vi "メイン.vi"() -> (2 "測定周期/ms":dbl, 3 "値転記用配列":T2[](array[typedef]))   [LabVIEW 2021] (continued)
                                w445 = FALSE
                                n187 = property on="メイン測定ボタン_単発 1" class="Bool (指定)"("Visible"=w445) -> ()  [unwired: 2 in, 2 out]
                                n188 = property on="メイン測定ボタン_連続 1" class="Bool (指定)"("Visible"=w445) -> ()  [unwired: 2 in, 2 out]
                              }
                              frame True {
                              }
                            }
                            n189 = local read "メインON/OFF_\n設定 1"() -> (w442:T1)
                            n190 = local write "メインON/OFF_\n保存確認 1"(w442) -> ()
                            n191 = local write "メインON/OFF_制御器 1"(w442) -> ()
                            n192 = property on="メインON/OFF_制御器" class="Clust (指定)"("Visible"=w439) -> ()  [unwired: 2 in, 2 out]
                            n193 = property on="メイン設定No_設定" class="Clust (指定)"("Visible"=w439) -> ()  [unwired: 2 in, 2 out]
                            n194 = property on="メイン設定_設定" class="Clust (指定)"("Visible"=w439) -> ()  [unwired: 2 in, 2 out]
                            n195 = property on="キャンセルボタン" class="Bool (指定)"("Visible"=w439) -> ()  [unwired: 2 in, 2 out]
                          }
                        }
                        n196 = global write "測定キャンセルボタン.vi" "グローバル_測定キャンセルボタン"(w98) -> ()
                        n197 = local write "G_メイン測定キャンセルボタン"(w98) -> ()
                        n198 = local write "測定旧値 1"(w98) -> ()
                        n199 = local write "測定新値 1"(w98) -> ()
                        n200 = control-ref of="このVI"() -> (w95:refnum<vi>)
                        n201 = Unbundle(w97) -> ("Vertical"=w96:i16)  [unwired: 1 out]
                        n202 = Replace Array Subset(array=w101, new element=w100, index=0) -> (w102:T2[])
                        n203 = property on="ペーン 2" class="Pane"("Origin"=w97) -> ()  [unwired: 2 in, 2 out]
                        n204 = call "メイン_装飾移動サブ.vi"("Y軸座標入力"=w96, "VI入力"=w95) -> ()  [unwired: 10 in]
                      }
                    }
                  }
                }
                frame 1 {
                  # "⑱"
                  # "⑰"
                  # "2つ目の配列に転記"
                  # "32回繰り返す為、増やす場合はこのケースストラクチャーを複製する\n複製時、設定項目の配列やボタンも複製する為、下記のボタン類の移動はしない事"
                  # "iniからデータ読み取り"
                  n205 = flat-sequence {
                    tunnel: w456 -> [w482]
                    tunnel: w455 -> [w483]
                    tunnel: [w461] -> w452
                    tunnel: [w460] -> w451
                    tunnel: w452 -> [w629]
                    tunnel: w451 -> [w628]
                    tunnel: [w629] -> w450
                    tunnel: [w628] -> w449
                    tunnel: [w676] -> w457
                    tunnel: [w677] -> w458
                    tunnel: w450 -> [w677]
                    tunnel: w449 -> [w676]
                    tunnel: [w673] -> w447
                    frame #0 {
                      w459 = "設定2"
                      # "複製時に変更する項目\n①②③④⑤⑥⑦⑧⑨　⑪⑫\nローカル変数\n⑬⑭\nセレクション\n⑮⑯\nプロパティノードが\n対象配列になっているか確認\n⑰\n指標値\n⑱\n複製したケースのTrue定数を削除"
                      # "⑭"
                      # "⑬"
                      # "⑫"
                      # "⑪"
                      # "④"
                      # "③"
                      # "setting.iniファイルからの設定項目の読み取り"
                      n206 = local read "メイン設定No_設定 2"() -> (w479:T5)
                      n207 = call-poly <vilib>:"Read Key.vi"("section"="No2.", "error in (no error)"=w483, "key"="No.", "refnum"=w482) -> ("error out"=w476:errorcluster, "value"=w480:i32, "refnum out"=w474:T10)  [unwired: 4 in, 1 out]
                      n208 = Bundle By Name(cluster=w479, "No."=w480) -> (w481:T5)
                      n209 = local write "メイン設定No_設定 2"(w481) -> ()
                      n210 = for {
                        shift-right: [w491] -> w478
                        shift-left: w474 -> [w492]
                        shift-right: [w488] -> w477
                        shift-left: w476 -> [w489]
                        tunnel: string[] ["規格", "規格上限", "規格下限", "ポートNo.", "測定モード", "規格単位", "品質チェック項目", "測定周期", "実測MAX", "実測MIN", "実測(MAX)", "実測(MIN)", "測定画面表示ボタン", "ゲージポートNo."] -> [w487] mode=indexing
                        tunnel: w459 -> [w484]
                        i -> [w490]
                        # "②"
                        # "①"
                        n211 = local read "メイン設定_設定 2"() -> (w485:T2)
                        n212 = case shown="0, デフォルト" w490 {
                          tunnel: w492 -> [w501 w510 w519 w528 w537 w546 w555 w564 w573 w582 w591 w600 w609 w618]
                          tunnel: [w500 w509 w518 w527 w536 w545 w554 w563 w572 w581 w590 w599 w608 w617] -> w491
                          tunnel: w484 -> [w499 w508 w517 w526 w535 w544 w553 w562 w571 w580 w589 w598 w607 w616]
                          tunnel: w489 -> [w498 w507 w516 w525 w534 w543 w552 w561 w570 w579 w588 w597 w606 w615]
                          tunnel: [w497 w506 w515 w524 w533 w542 w551 w560 w569 w578 w587 w596 w605 w614] -> w488
                          tunnel: w487 -> [_ _ _ _ _ w540 _ _ _ _ _ _ _ _]
                          tunnel: w487 -> [_ _ _ _ _ _ w549 _ _ _ _ w594 _ _]
                          tunnel: w487 -> [w495 w504 w513 w522 w531 _ _ w558 w567 w576 w585 _ w603 w612]
                          tunnel: [w494 w503 w512 w521 w530 w538 w547 w556 w566 w575 w584 w593 w602 w611] -> w486
                          tunnel: w485 -> [w493 w502 w511 w520 w529 w539 w548 w557 w565 w574 w583 w592 w601 w610]
                          frame 0, Default {
                            n213 = call-poly <vilib>:"Read Key.vi"("section"=w499, "error in (no error)"=w498, "key"=w495, "refnum"=w501) -> ("error out"=w497:errorcluster, "value"=w496:string, "refnum out"=w500:T10)  [unwired: 4 in, 1 out]
                            n214 = Bundle By Name(cluster=w493, "規格"=w496) -> (w494:T2)
                          }
                          frame 1 {
                            n215 = call-poly <vilib>:"Read Key.vi"("section"=w508, "error in (no error)"=w507, "key"=w504, "refnum"=w510) -> ("error out"=w506:errorcluster, "value"=w505:string, "refnum out"=w509:T10)  [unwired: 4 in, 1 out]
                            n216 = Bundle By Name(cluster=w502, "規格上限"=w505) -> (w503:T2)
                          }
                          frame 2 {
                            n217 = call-poly <vilib>:"Read Key.vi"("section"=w517, "error in (no error)"=w516, "key"=w513, "refnum"=w519) -> ("error out"=w515:errorcluster, "value"=w514:string, "refnum out"=w518:T10)  [unwired: 4 in, 1 out]
                            n218 = Bundle By Name(cluster=w511, "規格下限"=w514) -> (w512:T2)
                          }
                          frame 3 {
                            n219 = call-poly <vilib>:"Read Key.vi"("section"=w526, "error in (no error)"=w525, "key"=w522, "refnum"=w528) -> ("error out"=w524:errorcluster, "value"=w523:i32, "refnum out"=w527:T10)  [unwired: 4 in, 1 out]
                            n220 = Bundle By Name(cluster=w520, "ポートNo."=w523) -> (w521:T2)
                          }
                          frame 4 {
                            n221 = call-poly <vilib>:"Read Key.vi"("section"=w535, "error in (no error)"=w534, "key"=w531, "refnum"=w537) -> ("error out"=w533:errorcluster, "value"=w532:i32, "refnum out"=w536:T10)  [unwired: 4 in, 1 out]
                            n222 = Bundle By Name(cluster=w529, "測定モード"=w532) -> (w530:T2)
                          }
                          frame 5 {
                            n223 = call-poly <vilib>:"Read Key.vi"("section"=w544, "error in (no error)"=w543, "key"=w540, "refnum"=w546) -> ("error out"=w542:errorcluster, "value"=w541:string, "refnum out"=w545:T10)  [unwired: 4 in, 1 out]
                            n224 = Bundle By Name(cluster=w539, "規格単位"=w541) -> (w538:T2)
                          }
                          frame 6 {
                            n225 = call-poly <vilib>:"Read Key.vi"("section"=w553, "error in (no error)"=w552, "key"=w549, "refnum"=w555) -> ("error out"=w551:errorcluster, "value"=w550:string, "refnum out"=w554:T10)  [unwired: 4 in, 1 out]
                            n226 = Bundle By Name(cluster=w548, "品質チェック項目"=w550) -> (w547:T2)
                          }
                          frame 7 {
                            n227 = call-poly <vilib>:"Read Key.vi"("section"=w562, "error in (no error)"=w561, "key"=w558, "refnum"=w564) -> ("error out"=w560:errorcluster, "value"=w559:i32, "refnum out"=w563:T10)  [unwired: 4 in, 1 out]
                            n228 = Bundle By Name(cluster=w557, "測定周期"=w559) -> (w556:T2)
                          }
                          frame 8 {
                            n229 = call-poly <vilib>:"Read Key.vi"("section"=w571, "error in (no error)"=w570, "key"=w567, "refnum"=w573) -> ("error out"=w569:errorcluster, "value"=w568:string, "refnum out"=w572:T10)  [unwired: 4 in, 1 out]
                            n230 = Bundle By Name(cluster=w565, "実測値MAX"=w568) -> (w566:T2)
                          }
                          frame 9 {
                            n231 = call-poly <vilib>:"Read Key.vi"("section"=w580, "error in (no error)"=w579, "key"=w576, "refnum"=w582) -> ("error out"=w578:errorcluster, "value"=w577:string, "refnum out"=w581:T10)  [unwired: 4 in, 1 out]
                            n232 = Bundle By Name(cluster=w574, "実測値MIN"=w577) -> (w575:T2)
                          }
                          frame 10 {
                            n233 = call-poly <vilib>:"Read Key.vi"("section"=w589, "error in (no error)"=w588, "key"=w585, "refnum"=w591) -> ("error out"=w587:errorcluster, "value"=w586:string, "refnum out"=w590:T10)  [unwired: 4 in, 1 out]
                            n234 = Bundle By Name(cluster=w583, "実測値(MAX)"=w586) -> (w584:T2)
                          }
                          frame 11 {
                            n235 = call-poly <vilib>:"Read Key.vi"("section"=w598, "error in (no error)"=w597, "key"=w594, "refnum"=w600) -> ("error out"=w596:errorcluster, "value"=w595:string, "refnum out"=w599:T10)  [unwired: 4 in, 1 out]
                            n236 = Bundle By Name(cluster=w592, "実測値(MIN)"=w595) -> (w593:T2)
                          }
                          frame 12 {
                            n237 = call-poly <vilib>:"Read Key.vi"("section"=w607, "error in (no error)"=w606, "key"=w603, "refnum"=w609) -> ("error out"=w605:errorcluster, "value"=w604:bool, "refnum out"=w608:T10)  [unwired: 4 in, 1 out]
                            n238 = Bundle By Name(cluster=w601, "測定画面表示ボタン"=w604) -> (w602:T2)
                          }
                          frame 13 {
                            n239 = call-poly <vilib>:"Read Key.vi"("section"=w616, "error in (no error)"=w615, "key"=w612, "refnum"=w618) -> ("error out"=w614:errorcluster, "value"=w613:string, "refnum out"=w617:T10)  [unwired: 4 in, 1 out]
                            n240 = Bundle By Name(cluster=w610, "ゲージポートNo"=w613) -> (w611:T2)
                          }
                        }
                        n241 = local write "メイン設定_設定 2"(w486) -> ()
                      }
                      n242 = local read "メインON/OFF_\n設定 2"() -> (w470:T1)
                      n243 = call-poly <vilib>:"Read Key.vi"("section"=w459, "error in (no error)"=w477, "key"="使用ON/OFF", "refnum"=w478) -> ("error out"=w465:errorcluster, "value"=w468:bool, "refnum out"=w466:T10)  [unwired: 4 in, 1 out]
                      n244 = Bundle By Name(cluster=w470, "使用ON/OFF"=w468) -> (w471:T1)
                      n245 = local write "メインON/OFF_\n設定 2"(w471) -> ()
                      n246 = local read "CSV項目名 2"() -> (w464:T3)
                      n247 = call-poly <vilib>:"Read Key.vi"("section"=w459, "error in (no error)"=w465, "key"="CSVヘッダー名", "refnum"=w466) -> ("error out"=w460:errorcluster, "value"=w462:string, "refnum out"=w461:T10)  [unwired: 4 in, 1 out]
                      n248 = Bundle By Name(cluster=w464, "CSV項目名"=w462) -> (w463:T3)
                      n249 = local write "CSV項目名 2"(w463) -> ()
                    }
                    frame #1 {
                      # "csvヘッダー項目作成"
                      # "⑮"
                      # "⑤"
                      n250 = local read "CSV項目名 2"() -> (w623:T3)
                      n251 = Unbundle By Name(w623) -> ("CSV項目名"=w620:string)
                      n252 = local read "メイン設定_設定 2"() -> (w624:T2)
                      n253 = Unbundle By Name(w624) -> ("測定モード"=w619:u16)
                      n254 = case shown="0, デフォルト" w619 {
                        tunnel: ["単発測定" _ "多点測定"] -> w627
                        tunnel: [FALSE TRUE FALSE] -> w626
                        tunnel: [TRUE FALSE TRUE] -> w625
                        frame 0, Default {
                        }
                        frame 1 {
                        }
                        frame 2 {
                        }
                      }
                      n255 = case shown="1" w619 {
                        tunnel: w620 -> [w633 w645 w654]
                        tunnel: [w631 w643 w656] -> w622
                        tunnel: [w630 w642 w655] -> w621
                        frame 1 {
                          n256 = Empty String/Path?(string/path=w633) -> (empty?=w632:bool)
                          n257 = case shown="FALSE" w632 {
                            tunnel: w633 -> [w639 _]
                            tunnel: w633 -> [w638 _]
                            tunnel: [w635 ""] -> w631
                            tunnel: [w634 ""] -> w630
                            frame False {
                              n258 = Concatenate Strings(w639, "_max") -> (w635:string)
                              n259 = Concatenate Strings(w638, "_min") -> (w634:string)
                            }
                            frame True {
                            }
                          }
                        }
                        frame 2 {
                          n260 = Empty String/Path?(string/path=w645) -> (empty?=w644:bool)
                          n261 = case shown="FALSE" w644 {
                            tunnel: w645 -> [w651 _]
                            tunnel: w645 -> [w650 _]
                            tunnel: [w647 ""] -> w643
                            tunnel: [w646 ""] -> w642
                            frame False {
                              n262 = Concatenate Strings(w651, "_max") -> (w647:string)
                              n263 = Concatenate Strings(w650, "_min") -> (w646:string)
                            }
                            frame True {
                            }
                          }
                        }
                        frame 0, Default {
                          n264 = Empty String/Path?(string/path=w654) -> (empty?=w657:bool)
                          n265 = case shown="FALSE" w657 {
                            tunnel: w654 -> [w661 _]
                            tunnel: [w659 ""] -> w656
                            tunnel: ["" ""] -> w655
                            frame False {
                              n266 = Concatenate Strings(w661, "_value") -> (w659:string)
                            }
                            frame True {
                            }
                          }
                        }
                      }
                      n267 = property on="メイン測定ボタン_単発 2" class="Bool (指定)"("BoolText.Text"=w627) -> ()  [unwired: 2 in, 2 out]
                      n268 = local write "csv入力項目min 2"(w621) -> ()
                      n269 = local write "csv入力項目max 2"(w622) -> ()
                      n270 = property on="メイン測定ボタン_連続 2" class="Bool (指定)"("Visible"=w626) -> ()  [unwired: 2 in, 2 out]
                      n271 = property on="メイン測定ボタン_単発 2" class="Bool (指定)"("Visible"=w625) -> ()  [unwired: 2 in, 2 out]
                    }
                    frame #2 {
                      # "⑯"
                      # "⑨"
                      # "⑧"
                      # "⑦"
                      # "⑥"
                      n272 = local read "メインON/OFF_\n設定 2"() -> (w675:T1)
                      n273 = local write "メインON/OFF_\n保存確認 2"(w675) -> ()
                      n274 = local read "メイン設定_設定 2"() -> (w673:T2)
                      n275 = Unbundle By Name(w673) -> ("測定画面表示ボタン"=w672:bool)
                      n276 = case shown="FALSE" w672 {
                        tunnel: [w678 TRUE] -> w674
                        frame False {
                          w678 = FALSE
                          n277 = property on="メイン測定ボタン_単発 2" class="Bool (指定)"("Visible"=w678) -> ()  [unwired: 2 in, 2 out]
                          n278 = property on="メイン測定ボタン_連続 2" class="Bool (指定)"("Visible"=w678) -> ()  [unwired: 2 in, 2 out]
                        }
                        frame True {
                        }
                      }
                      n279 = local write "メインON/OFF_制御器 2"(w675) -> ()
                      n280 = property on="メインON/OFF_制御器 2" class="Clust (指定)"("Visible"=w674) -> ()  [unwired: 2 in, 2 out]
                      n281 = property on="メイン設定No_設定 2" class="Clust (指定)"("Visible"=w674) -> ()  [unwired: 2 in, 2 out]
                      n282 = property on="メイン設定_設定 2" class="Clust (指定)"("Visible"=w674) -> ()  [unwired: 2 in, 2 out]
                      n283 = property on="キャンセルボタン 2" class="Bool (指定)"("Visible"=w674) -> ()  [unwired: 2 in, 2 out]
                    }
                  }
                  n284 = Replace Array Subset(array=w454, new element=w447, index=1) -> (w453:T2[])
                }
                frame 2 {
                  # "⑱"
                  # "⑰"
                  # "2つ目の配列に転記"
                  # "32回繰り返す為、増やす場合はこのケースストラクチャーを複製する\n複製時、設定項目の配列やボタンも複製する為、下記のボタン類の移動はしない事"
                  # "iniからデータ読み取り"
                  n285 = flat-sequence {
                    tunnel: w689 -> [w715]
                    tunnel: w688 -> [w716]
                    tunnel: [w693] -> w685
                    tunnel: [w694] -> w684
                    tunnel: w685 -> [w862]
                    tunnel: w684 -> [w861]
                    tunnel: [w862] -> w683
                    tunnel: [w861] -> w682
                    tunnel: [w909] -> w690
                    tunnel: [w910] -> w691
                    tunnel: w683 -> [w910]
                    tunnel: w682 -> [w909]
                    tunnel: [w906] -> w680
                    frame #0 {
                      w692 = "設定3"
                      # "複製時に変更する項目\n①②③④⑤⑥⑦⑧⑨　⑪⑫\nローカル変数\n⑬⑭\nセレクション\n⑮⑯\nプロパティノードが\n対象配列になっているか確認\n⑰\n指標値\n⑱\n複製したケースのTrue定数を削除"
                      # "⑭"
                      # "⑬"
                      # "⑫"
                      # "⑪"
                      # "④"
                      # "③"
                      # "setting.iniファイルからの設定項目の読み取り"
                      n286 = local read "メイン設定No_設定 3"() -> (w712:T5)
                      n287 = call-poly <vilib>:"Read Key.vi"("section"="No3.", "error in (no error)"=w716, "key"="No.", "refnum"=w715) -> ("error out"=w709:errorcluster, "value"=w713:i32, "refnum out"=w707:T10)  [unwired: 4 in, 1 out]
                      n288 = Bundle By Name(cluster=w712, "No."=w713) -> (w714:T5)
                      n289 = local write "メイン設定No_設定 3"(w714) -> ()
                      n290 = for {
                        shift-right: [w724] -> w711
                        shift-left: w707 -> [w725]
                        shift-right: [w721] -> w710
                        shift-left: w709 -> [w722]
                        tunnel: string[] ["規格", "規格上限", "規格下限", "ポートNo.", "測定モード", "規格単位", "品質チェック項目", "測定周期", "実測MAX", "実測MIN", "実測(MAX)", "実測(MIN)", "測定画面表示ボタン", "ゲージポートNo."] -> [w720] mode=indexing
                        tunnel: w692 -> [w717]
                        i -> [w723]
                        # "②"
                        # "①"
                        n291 = local read "メイン設定_設定 3"() -> (w718:T2)
                        n292 = case shown="0, デフォルト" w723 {
                          tunnel: w725 -> [w734 w743 w752 w761 w770 w779 w788 w797 w806 w815 w824 w833 w842 w851]
                          tunnel: [w733 w742 w751 w760 w769 w778 w787 w796 w805 w814 w823 w832 w841 w850] -> w724
                          tunnel: w717 -> [w732 w741 w750 w759 w768 w777 w786 w795 w804 w813 w822 w831 w840 w849]
                          tunnel: w722 -> [w731 w740 w749 w758 w767 w776 w785 w794 w803 w812 w821 w830 w839 w848]
                          tunnel: [w730 w739 w748 w757 w766 w775 w784 w793 w802 w811 w820 w829 w838 w847] -> w721
                          tunnel: w720 -> [_ _ _ _ _ w773 _ _ _ _ _ _ _ _]
                          tunnel: w720 -> [_ _ _ _ _ _ w782 _ _ _ _ w827 _ _]
                          tunnel: w720 -> [w728 w737 w746 w755 w764 _ _ w791 w800 w809 w818 _ w836 w845]
                          tunnel: [w727 w736 w745 w754 w763 w771 w780 w789 w799 w808 w817 w826 w835 w844] -> w719
                          tunnel: w718 -> [w726 w735 w744 w753 w762 w772 w781 w790 w798 w807 w816 w825 w834 w843]
                          frame 0, Default {
                            n293 = call-poly <vilib>:"Read Key.vi"("section"=w732, "error in (no error)"=w731, "key"=w728, "refnum"=w734) -> ("error out"=w730:errorcluster, "value"=w729:string, "refnum out"=w733:T10)  [unwired: 4 in, 1 out]
                            n294 = Bundle By Name(cluster=w726, "規格"=w729) -> (w727:T2)
                          }
                          frame 1 {
                            n295 = call-poly <vilib>:"Read Key.vi"("section"=w741, "error in (no error)"=w740, "key"=w737, "refnum"=w743) -> ("error out"=w739:errorcluster, "value"=w738:string, "refnum out"=w742:T10)  [unwired: 4 in, 1 out]
                            n296 = Bundle By Name(cluster=w735, "規格上限"=w738) -> (w736:T2)
                          }
                          frame 2 {
                            n297 = call-poly <vilib>:"Read Key.vi"("section"=w750, "error in (no error)"=w749, "key"=w746, "refnum"=w752) -> ("error out"=w748:errorcluster, "value"=w747:string, "refnum out"=w751:T10)  [unwired: 4 in, 1 out]
                            n298 = Bundle By Name(cluster=w744, "規格下限"=w747) -> (w745:T2)
                          }
                          frame 3 {
                            n299 = call-poly <vilib>:"Read Key.vi"("section"=w759, "error in (no error)"=w758, "key"=w755, "refnum"=w761) -> ("error out"=w757:errorcluster, "value"=w756:i32, "refnum out"=w760:T10)  [unwired: 4 in, 1 out]
                            n300 = Bundle By Name(cluster=w753, "ポートNo."=w756) -> (w754:T2)
                          }
                          frame 4 {
                            n301 = call-poly <vilib>:"Read Key.vi"("section"=w768, "error in (no error)"=w767, "key"=w764, "refnum"=w770) -> ("error out"=w766:errorcluster, "value"=w765:i32, "refnum out"=w769:T10)  [unwired: 4 in, 1 out]
                            n302 = Bundle By Name(cluster=w762, "測定モード"=w765) -> (w763:T2)
                          }
                          frame 5 {
                            n303 = call-poly <vilib>:"Read Key.vi"("section"=w777, "error in (no error)"=w776, "key"=w773, "refnum"=w779) -> ("error out"=w775:errorcluster, "value"=w774:string, "refnum out"=w778:T10)  [unwired: 4 in, 1 out]
                            n304 = Bundle By Name(cluster=w772, "規格単位"=w774) -> (w771:T2)
                          }
                          frame 6 {
                            n305 = call-poly <vilib>:"Read Key.vi"("section"=w786, "error in (no error)"=w785, "key"=w782, "refnum"=w788) -> ("error out"=w784:errorcluster, "value"=w783:string, "refnum out"=w787:T10)  [unwired: 4 in, 1 out]
                            n306 = Bundle By Name(cluster=w781, "品質チェック項目"=w783) -> (w780:T2)
                          }
                          frame 7 {
                            n307 = call-poly <vilib>:"Read Key.vi"("section"=w795, "error in (no error)"=w794, "key"=w791, "refnum"=w797) -> ("error out"=w793:errorcluster, "value"=w792:i32, "refnum out"=w796:T10)  [unwired: 4 in, 1 out]
                            n308 = Bundle By Name(cluster=w790, "測定周期"=w792) -> (w789:T2)
                          }
                          frame 8 {
                            n309 = call-poly <vilib>:"Read Key.vi"("section"=w804, "error in (no error)"=w803, "key"=w800, "refnum"=w806) -> ("error out"=w802:errorcluster, "value"=w801:string, "refnum out"=w805:T10)  [unwired: 4 in, 1 out]
                            n310 = Bundle By Name(cluster=w798, "実測値MAX"=w801) -> (w799:T2)
                          }
                          frame 9 {
                            n311 = call-poly <vilib>:"Read Key.vi"("section"=w813, "error in (no error)"=w812, "key"=w809, "refnum"=w815) -> ("error out"=w811:errorcluster, "value"=w810:string, "refnum out"=w814:T10)  [unwired: 4 in, 1 out]
                            n312 = Bundle By Name(cluster=w807, "実測値MIN"=w810) -> (w808:T2)
                          }
                          frame 10 {
                            n313 = call-poly <vilib>:"Read Key.vi"("section"=w822, "error in (no error)"=w821, "key"=w818, "refnum"=w824) -> ("error out"=w820:errorcluster, "value"=w819:string, "refnum out"=w823:T10)  [unwired: 4 in, 1 out]
                            n314 = Bundle By Name(cluster=w816, "実測値(MAX)"=w819) -> (w817:T2)
                          }
                          frame 11 {
                            n315 = call-poly <vilib>:"Read Key.vi"("section"=w831, "error in (no error)"=w830, "key"=w827, "refnum"=w833) -> ("error out"=w829:errorcluster, "value"=w828:string, "refnum out"=w832:T10)  [unwired: 4 in, 1 out]
                            n316 = Bundle By Name(cluster=w825, "実測値(MIN)"=w828) -> (w826:T2)
                          }
                          frame 12 {
                            n317 = call-poly <vilib>:"Read Key.vi"("section"=w840, "error in (no error)"=w839, "key"=w836, "refnum"=w842) -> ("error out"=w838:errorcluster, "value"=w837:bool, "refnum out"=w841:T10)  [unwired: 4 in, 1 out]
                            n318 = Bundle By Name(cluster=w834, "測定画面表示ボタン"=w837) -> (w835:T2)
                          }
                          frame 13 {
                            n319 = call-poly <vilib>:"Read Key.vi"("section"=w849, "error in (no error)"=w848, "key"=w845, "refnum"=w851) -> ("error out"=w847:errorcluster, "value"=w846:string, "refnum out"=w850:T10)  [unwired: 4 in, 1 out]
                            n320 = Bundle By Name(cluster=w843, "ゲージポートNo"=w846) -> (w844:T2)
                          }
                        }
                        n321 = local write "メイン設定_設定 3"(w719) -> ()
                      }
                      n322 = local read "メインON/OFF_\n設定 3"() -> (w703:T1)
                      n323 = call-poly <vilib>:"Read Key.vi"("section"=w692, "error in (no error)"=w710, "key"="使用ON/OFF", "refnum"=w711) -> ("error out"=w695:errorcluster, "value"=w701:bool, "refnum out"=w696:T10)  [unwired: 4 in, 1 out]
                      n324 = Bundle By Name(cluster=w703, "使用ON/OFF"=w701) -> (w704:T1)
                      n325 = local write "メインON/OFF_\n設定 3"(w704) -> ()
                      n326 = local read "CSV項目名 3"() -> (w699:T3)
                      n327 = call-poly <vilib>:"Read Key.vi"("section"=w692, "error in (no error)"=w695, "key"="CSVヘッダー名", "refnum"=w696) -> ("error out"=w694:errorcluster, "value"=w697:string, "refnum out"=w693:T10)  [unwired: 4 in, 1 out]
                      n328 = Bundle By Name(cluster=w699, "CSV項目名"=w697) -> (w698:T3)
                      n329 = local write "CSV項目名 3"(w698) -> ()
                    }
                    frame #1 {
                      # "csvヘッダー項目作成"
                      # "⑮"
                      # "⑤"
                      n330 = local read "CSV項目名 3"() -> (w856:T3)
                      n331 = Unbundle By Name(w856) -> ("CSV項目名"=w853:string)
                      n332 = local read "メイン設定_設定 3"() -> (w857:T2)
                      n333 = Unbundle By Name(w857) -> ("測定モード"=w852:u16)
                      n334 = case shown="0, デフォルト" w852 {
                        tunnel: ["単発測定" _ "多点測定"] -> w860
                        tunnel: [FALSE TRUE FALSE] -> w859
                        tunnel: [TRUE FALSE TRUE] -> w858
                        frame 0, Default {
                        }
                        frame 1 {
                        }
                        frame 2 {
                        }
                      }
                      n335 = case shown="1" w852 {
                        tunnel: w853 -> [w866 w878 w887]
                        tunnel: [w864 w876 w889] -> w855
                        tunnel: [w863 w875 w888] -> w854
                        frame 1 {
                          n336 = Empty String/Path?(string/path=w866) -> (empty?=w865:bool)
                          n337 = case shown="FALSE" w865 {
                            tunnel: w866 -> [w872 _]
                            tunnel: w866 -> [w871 _]
                            tunnel: [w868 ""] -> w864
                            tunnel: [w867 ""] -> w863
                            frame False {
                              n338 = Concatenate Strings(w872, "_max") -> (w868:string)
                              n339 = Concatenate Strings(w871, "_min") -> (w867:string)
                            }
                            frame True {
                            }
                          }
                        }
                        frame 2 {
                          n340 = Empty String/Path?(string/path=w878) -> (empty?=w877:bool)
                          n341 = case shown="FALSE" w877 {
                            tunnel: w878 -> [w884 _]
                            tunnel: w878 -> [w883 _]
                            tunnel: [w880 ""] -> w876
                            tunnel: [w879 ""] -> w875
                            frame False {
                              n342 = Concatenate Strings(w884, "_max") -> (w880:string)
                              n343 = Concatenate Strings(w883, "_min") -> (w879:string)
                            }
                            frame True {
                            }
                          }
                        }
                        frame 0, Default {
                          n344 = Empty String/Path?(string/path=w887) -> (empty?=w890:bool)
                          n345 = case shown="FALSE" w890 {
                            tunnel: w887 -> [w894 _]
                            tunnel: [w892 ""] -> w889
                            tunnel: ["" ""] -> w888
                            frame False {
                              n346 = Concatenate Strings(w894, "_value") -> (w892:string)
                            }
                            frame True {
                            }
                          }
                        }
                      }
                      n347 = property on="メイン測定ボタン_単発 3" class="Bool (指定)"("BoolText.Text"=w860) -> ()  [unwired: 2 in, 2 out]
                      n348 = local write "csv入力項目min 3"(w854) -> ()
                      n349 = local write "csv入力項目max 3"(w855) -> ()
                      n350 = property on="メイン測定ボタン_連続 3" class="Bool (指定)"("Visible"=w859) -> ()  [unwired: 2 in, 2 out]
                      n351 = property on="メイン測定ボタン_単発 3" class="Bool (指定)"("Visible"=w858) -> ()  [unwired: 2 in, 2 out]
                    }
                    frame #2 {
                      # "⑯"
                      # "⑨"
                      # "⑧"
                      # "⑦"
                      # "⑥"
                      n352 = local read "メインON/OFF_\n設定 3"() -> (w908:T1)
                      n353 = local write "メインON/OFF_\n保存確認 3"(w908) -> ()
                      n354 = local read "メイン設定_設定 3"() -> (w906:T2)
                      n355 = Unbundle By Name(w906) -> ("測定画面表示ボタン"=w905:bool)
                      n356 = case shown="FALSE" w905 {
                        tunnel: [w911 TRUE] -> w907
                        frame False {
                          w911 = FALSE
                          n357 = property on="メイン測定ボタン_単発 3" class="Bool (指定)"("Visible"=w911) -> ()  [unwired: 2 in, 2 out]
                          n358 = property on="メイン測定ボタン_連続 3" class="Bool (指定)"("Visible"=w911) -> ()  [unwired: 2 in, 2 out]
                        }
                        frame True {
                        }
                      }
                      n359 = local write "メインON/OFF_制御器 3"(w908) -> ()
                      n360 = property on="メインON/OFF_制御器 3" class="Clust (指定)"("Visible"=w907) -> ()  [unwired: 2 in, 2 out]
                      n361 = property on="メイン設定No_設定 3" class="Clust (指定)"("Visible"=w907) -> ()  [unwired: 2 in, 2 out]
                      n362 = property on="メイン設定_設定 3" class="Clust (指定)"("Visible"=w907) -> ()  [unwired: 2 in, 2 out]
                      n363 = property on="キャンセルボタン 3" class="Bool (指定)"("Visible"=w907) -> ()  [unwired: 2 in, 2 out]
                    }
                  }
                  n364 = Replace Array Subset(array=w687, new element=w680, index=2) -> (w686:T2[])
                }
                frame 3 {
                  # "⑱"
                  # "⑰"
                  # "2つ目の配列に転記"
                  # "32回繰り返す為、増やす場合はこのケースストラクチャーを複製する\n複製時、設定項目の配列やボタンも複製する為、下記のボタン類の移動はしない事"
                  # "iniからデータ読み取り"
                  n365 = flat-sequence {
                    tunnel: w922 -> [w948]
                    tunnel: w921 -> [w949]
                    tunnel: [w927] -> w918
                    tunnel: [w926] -> w913
                    tunnel: w918 -> [w1095]
                    tunnel: [w1095] -> w917
                    tunnel: [w1094] -> w916
                    tunnel: w913 -> [w1094]
                    tunnel: [w1142] -> w923
                    tunnel: [w1143] -> w924
                    tunnel: w917 -> [w1143]
                    tunnel: w916 -> [w1142]
                    tunnel: [w1139] -> w914
                    frame #0 {
                      w925 = "設定4"
                      # "複製時に変更する項目\n①②③④⑤⑥⑦⑧⑨　⑪⑫\nローカル変数\n⑬⑭\nセレクション\n⑮⑯\nプロパティノードが\n対象配列になっているか確認\n⑰\n指標値\n⑱\n複製したケースのTrue定数を削除"
                      # "⑭"
                      # "⑬"
                      # "⑫"
                      # "⑪"
                      # "④"
                      # "③"
                      # "setting.iniファイルからの設定項目の読み取り"
                      n366 = local read "メイン設定No_設定 4"() -> (w945:T5)
                      n367 = call-poly <vilib>:"Read Key.vi"("section"="No4.", "error in (no error)"=w949, "key"="No.", "refnum"=w948) -> ("error out"=w942:errorcluster, "value"=w946:i32, "refnum out"=w940:T10)  [unwired: 4 in, 1 out]
                      n368 = Bundle By Name(cluster=w945, "No."=w946) -> (w947:T5)
                      n369 = local write "メイン設定No_設定 4"(w947) -> ()
                      n370 = for {
                        shift-right: [w957] -> w944
                        shift-left: w940 -> [w958]
                        shift-right: [w954] -> w943
                        shift-left: w942 -> [w955]
                        tunnel: string[] ["規格", "規格上限", "規格下限", "ポートNo.", "測定モード", "規格単位", "品質チェック項目", "測定周期", "実測MAX", "実測MIN", "実測(MAX)", "実測(MIN)", "測定画面表示ボタン", "ゲージポートNo."] -> [w953] mode=indexing
                        tunnel: w925 -> [w950]
                        i -> [w956]
                        # "②"
                        # "①"
                        n371 = local read "メイン設定_設定 4"() -> (w951:T2)
                        n372 = case shown="0, デフォルト" w956 {
                          tunnel: w958 -> [w967 w976 w985 w994 w1003 w1012 w1021 w1030 w1039 w1048 w1057 w1066 w1075 w1084]
                          tunnel: [w966 w975 w984 w993 w1002 w1011 w1020 w1029 w1038 w1047 w1056 w1065 w1074 w1083] -> w957
                          tunnel: w950 -> [w965 w974 w983 w992 w1001 w1010 w1019 w1028 w1037 w1046 w1055 w1064 w1073 w1082]
                          tunnel: w955 -> [w964 w973 w982 w991 w1000 w1009 w1018 w1027 w1036 w1045 w1054 w1063 w1072 w1081]
                          tunnel: [w963 w972 w981 w990 w999 w1008 w1017 w1026 w1035 w1044 w1053 w1062 w1071 w1080] -> w954
                          tunnel: w953 -> [_ _ _ _ _ w1006 _ _ _ _ _ _ _ _]
                          tunnel: w953 -> [_ _ _ _ _ _ w1015 _ _ _ _ w1060 _ _]
                          tunnel: w953 -> [w961 w970 w979 w988 w997 _ _ w1024 w1033 w1042 w1051 _ w1069 w1078]
                          tunnel: [w960 w969 w978 w987 w996 w1004 w1013 w1022 w1032 w1041 w1050 w1059 w1068 w1077] -> w952
                          tunnel: w951 -> [w959 w968 w977 w986 w995 w1005 w1014 w1023 w1031 w1040 w1049 w1058 w1067 w1076]
                          frame 0, Default {
                            n373 = call-poly <vilib>:"Read Key.vi"("section"=w965, "error in (no error)"=w964, "key"=w961, "refnum"=w967) -> ("error out"=w963:errorcluster, "value"=w962:string, "refnum out"=w966:T10)  [unwired: 4 in, 1 out]
                            n374 = Bundle By Name(cluster=w959, "規格"=w962) -> (w960:T2)
                          }
                          frame 1 {
                            n375 = call-poly <vilib>:"Read Key.vi"("section"=w974, "error in (no error)"=w973, "key"=w970, "refnum"=w976) -> ("error out"=w972:errorcluster, "value"=w971:string, "refnum out"=w975:T10)  [unwired: 4 in, 1 out]
                            n376 = Bundle By Name(cluster=w968, "規格上限"=w971) -> (w969:T2)
                          }
                          frame 2 {
                            n377 = call-poly <vilib>:"Read Key.vi"("section"=w983, "error in (no error)"=w982, "key"=w979, "refnum"=w985) -> ("error out"=w981:errorcluster, "value"=w980:string, "refnum out"=w984:T10)  [unwired: 4 in, 1 out]
                            n378 = Bundle By Name(cluster=w977, "規格下限"=w980) -> (w978:T2)
                          }
                          frame 3 {
                            n379 = call-poly <vilib>:"Read Key.vi"("section"=w992, "error in (no error)"=w991, "key"=w988, "refnum"=w994) -> ("error out"=w990:errorcluster, "value"=w989:i32, "refnum out"=w993:T10)  [unwired: 4 in, 1 out]
                            n380 = Bundle By Name(cluster=w986, "ポートNo."=w989) -> (w987:T2)
                          }
                          frame 4 {
                            n381 = call-poly <vilib>:"Read Key.vi"("section"=w1001, "error in (no error)"=w1000, "key"=w997, "refnum"=w1003) -> ("error out"=w999:errorcluster, "value"=w998:i32, "refnum out"=w1002:T10)  [unwired: 4 in, 1 out]
                            n382 = Bundle By Name(cluster=w995, "測定モード"=w998) -> (w996:T2)
                          }
                          frame 5 {
                            n383 = call-poly <vilib>:"Read Key.vi"("section"=w1010, "error in (no error)"=w1009, "key"=w1006, "refnum"=w1012) -> ("error out"=w1008:errorcluster, "value"=w1007:string, "refnum out"=w1011:T10)  [unwired: 4 in, 1 out]
                            n384 = Bundle By Name(cluster=w1005, "規格単位"=w1007) -> (w1004:T2)
                          }
                          frame 6 {
                            n385 = call-poly <vilib>:"Read Key.vi"("section"=w1019, "error in (no error)"=w1018, "key"=w1015, "refnum"=w1021) -> ("error out"=w1017:errorcluster, "value"=w1016:string, "refnum out"=w1020:T10)  [unwired: 4 in, 1 out]
                            n386 = Bundle By Name(cluster=w1014, "品質チェック項目"=w1016) -> (w1013:T2)
                          }
                          frame 7 {
                            n387 = call-poly <vilib>:"Read Key.vi"("section"=w1028, "error in (no error)"=w1027, "key"=w1024, "refnum"=w1030) -> ("error out"=w1026:errorcluster, "value"=w1025:i32, "refnum out"=w1029:T10)  [unwired: 4 in, 1 out]
                            n388 = Bundle By Name(cluster=w1023, "測定周期"=w1025) -> (w1022:T2)
                          }
                          frame 8 {
                            n389 = call-poly <vilib>:"Read Key.vi"("section"=w1037, "error in (no error)"=w1036, "key"=w1033, "refnum"=w1039) -> ("error out"=w1035:errorcluster, "value"=w1034:string, "refnum out"=w1038:T10)  [unwired: 4 in, 1 out]
                            n390 = Bundle By Name(cluster=w1031, "実測値MAX"=w1034) -> (w1032:T2)
                          }
                          frame 9 {
                            n391 = call-poly <vilib>:"Read Key.vi"("section"=w1046, "error in (no error)"=w1045, "key"=w1042, "refnum"=w1048) -> ("error out"=w1044:errorcluster, "value"=w1043:string, "refnum out"=w1047:T10)  [unwired: 4 in, 1 out]
                            n392 = Bundle By Name(cluster=w1040, "実測値MIN"=w1043) -> (w1041:T2)
                          }
                          frame 10 {
                            n393 = call-poly <vilib>:"Read Key.vi"("section"=w1055, "error in (no error)"=w1054, "key"=w1051, "refnum"=w1057) -> ("error out"=w1053:errorcluster, "value"=w1052:string, "refnum out"=w1056:T10)  [unwired: 4 in, 1 out]
                            n394 = Bundle By Name(cluster=w1049, "実測値(MAX)"=w1052) -> (w1050:T2)
                          }
                          frame 11 {
                            n395 = call-poly <vilib>:"Read Key.vi"("section"=w1064, "error in (no error)"=w1063, "key"=w1060, "refnum"=w1066) -> ("error out"=w1062:errorcluster, "value"=w1061:string, "refnum out"=w1065:T10)  [unwired: 4 in, 1 out]
                            n396 = Bundle By Name(cluster=w1058, "実測値(MIN)"=w1061) -> (w1059:T2)
                          }
                          frame 12 {
                            n397 = call-poly <vilib>:"Read Key.vi"("section"=w1073, "error in (no error)"=w1072, "key"=w1069, "refnum"=w1075) -> ("error out"=w1071:errorcluster, "value"=w1070:bool, "refnum out"=w1074:T10)  [unwired: 4 in, 1 out]
                            n398 = Bundle By Name(cluster=w1067, "測定画面表示ボタン"=w1070) -> (w1068:T2)
                          }
                          frame 13 {
                            n399 = call-poly <vilib>:"Read Key.vi"("section"=w1082, "error in (no error)"=w1081, "key"=w1078, "refnum"=w1084) -> ("error out"=w1080:errorcluster, "value"=w1079:string, "refnum out"=w1083:T10)  [unwired: 4 in, 1 out]
                            n400 = Bundle By Name(cluster=w1076, "ゲージポートNo"=w1079) -> (w1077:T2)
                          }
                        }
                        n401 = local write "メイン設定_設定 4"(w952) -> ()
                      }
                      n402 = local read "メインON/OFF_\n設定 4"() -> (w936:T1)
                      n403 = call-poly <vilib>:"Read Key.vi"("section"=w925, "error in (no error)"=w943, "key"="使用ON/OFF", "refnum"=w944) -> ("error out"=w928:errorcluster, "value"=w934:bool, "refnum out"=w929:T10)  [unwired: 4 in, 1 out]
                      n404 = Bundle By Name(cluster=w936, "使用ON/OFF"=w934) -> (w937:T1)
                      n405 = local write "メインON/OFF_\n設定 4"(w937) -> ()
                      n406 = local read "CSV項目名 4"() -> (w932:T3)
                      n407 = call-poly <vilib>:"Read Key.vi"("section"=w925, "error in (no error)"=w928, "key"="CSVヘッダー名", "refnum"=w929) -> ("error out"=w926:errorcluster, "value"=w930:string, "refnum out"=w927:T10)  [unwired: 4 in, 1 out]
                      n408 = Bundle By Name(cluster=w932, "CSV項目名"=w930) -> (w931:T3)
                      n409 = local write "CSV項目名 4"(w931) -> ()
                    }
                    frame #1 {
                      # "csvヘッダー項目作成"
                      # "⑮"
                      # "⑤"
                      n410 = local read "CSV項目名 4"() -> (w1089:T3)
                      n411 = Unbundle By Name(w1089) -> ("CSV項目名"=w1086:string)
                      n412 = local read "メイン設定_設定 4"() -> (w1090:T2)
                      n413 = Unbundle By Name(w1090) -> ("測定モード"=w1085:u16)
                      n414 = case shown="0, デフォルト" w1085 {
                        tunnel: ["単発測定" _ "多点測定"] -> w1093
                        tunnel: [FALSE TRUE FALSE] -> w1092
                        tunnel: [TRUE FALSE TRUE] -> w1091
                        frame 0, Default {
                        }
                        frame 1 {
                        }
                        frame 2 {
                        }
                      }
                      n415 = case shown="1" w1085 {
                        tunnel: w1086 -> [w1099 w1111 w1120]
                        tunnel: [w1097 w1109 w1122] -> w1088
                        tunnel: [w1096 w1108 w1121] -> w1087
                        frame 1 {
                          n416 = Empty String/Path?(string/path=w1099) -> (empty?=w1098:bool)
                          n417 = case shown="FALSE" w1098 {
                            tunnel: w1099 -> [w1105 _]
                            tunnel: w1099 -> [w1104 _]
                            tunnel: [w1101 ""] -> w1097
                            tunnel: [w1100 ""] -> w1096
                            frame False {
                              n418 = Concatenate Strings(w1105, "_max") -> (w1101:string)
                              n419 = Concatenate Strings(w1104, "_min") -> (w1100:string)
                            }
                            frame True {
                            }
                          }
                        }
                        frame 2 {
                          n420 = Empty String/Path?(string/path=w1111) -> (empty?=w1110:bool)
                          n421 = case shown="FALSE" w1110 {
                            tunnel: w1111 -> [w1117 _]
                            tunnel: w1111 -> [w1116 _]
                            tunnel: [w1113 ""] -> w1109
                            tunnel: [w1112 ""] -> w1108
                            frame False {
                              n422 = Concatenate Strings(w1117, "_max") -> (w1113:string)
                              n423 = Concatenate Strings(w1116, "_min") -> (w1112:string)
                            }
                            frame True {
                            }
                          }
                        }
                        frame 0, Default {
                          n424 = Empty String/Path?(string/path=w1120) -> (empty?=w1123:bool)
                          n425 = case shown="FALSE" w1123 {
                            tunnel: w1120 -> [w1127 _]
                            tunnel: [w1125 ""] -> w1122
                            tunnel: ["" ""] -> w1121
                            frame False {
                              n426 = Concatenate Strings(w1127, "_value") -> (w1125:string)
                            }
                            frame True {
                            }
                          }
                        }
                      }
                      n427 = property on="メイン測定ボタン_単発 4" class="Bool (指定)"("BoolText.Text"=w1093) -> ()  [unwired: 2 in, 2 out]
                      n428 = local write "csv入力項目min 4"(w1087) -> ()
                      n429 = local write "csv入力項目max 4"(w1088) -> ()
                      n430 = property on="メイン測定ボタン_連続 4" class="Bool (指定)"("Visible"=w1092) -> ()  [unwired: 2 in, 2 out]
                      n431 = property on="メイン測定ボタン_単発 4" class="Bool (指定)"("Visible"=w1091) -> ()  [unwired: 2 in, 2 out]
                    }
                    frame #2 {
                      # "⑯"
                      # "⑨"
                      # "⑧"
                      # "⑦"
                      # "⑥"
                      n432 = local read "メインON/OFF_\n設定 4"() -> (w1141:T1)
                      n433 = local write "メインON/OFF_\n保存確認 4"(w1141) -> ()
                      n434 = local read "メイン設定_設定 4"() -> (w1139:T2)
                      n435 = Unbundle By Name(w1139) -> ("測定画面表示ボタン"=w1138:bool)
                      n436 = case shown="FALSE" w1138 {
                        tunnel: [w1144 TRUE] -> w1140
                        frame False {
                          w1144 = FALSE
                          n437 = property on="メイン測定ボタン_単発 4" class="Bool (指定)"("Visible"=w1144) -> ()  [unwired: 2 in, 2 out]
                          n438 = property on="メイン測定ボタン_連続 4" class="Bool (指定)"("Visible"=w1144) -> ()  [unwired: 2 in, 2 out]
                        }
                        frame True {
                        }
                      }
                      n439 = local write "メインON/OFF_制御器 4"(w1141) -> ()
                      n440 = property on="メインON/OFF_制御器 4" class="Clust (指定)"("Visible"=w1140) -> ()  [unwired: 2 in, 2 out]
                      n441 = property on="メイン設定No_設定 4" class="Clust (指定)"("Visible"=w1140) -> ()  [unwired: 2 in, 2 out]
                      n442 = property on="メイン設定_設定 4" class="Clust (指定)"("Visible"=w1140) -> ()  [unwired: 2 in, 2 out]
                      n443 = property on="キャンセルボタン 4" class="Bool (指定)"("Visible"=w1140) -> ()  [unwired: 2 in, 2 out]
                    }
                  }
                  n444 = Replace Array Subset(array=w920, new element=w914, index=3) -> (w919:T2[])
                }
                frame 4 {
                  # "⑱"
                  # "⑰"
                  # "2つ目の配列に転記"
                  # "32回繰り返す為、増やす場合はこのケースストラクチャーを複製する\n複製時、設定項目の配列やボタンも複製する為、下記のボタン類の移動はしない事"
                  # "iniからデータ読み取り"
                  n445 = flat-sequence {
                    tunnel: w1155 -> [w1181]
                    tunnel: w1154 -> [w1182]
                    tunnel: [w1160] -> w1151
                    tunnel: [w1159] -> w1150
                    tunnel: w1151 -> [w1328]
                    tunnel: w1150 -> [w1327]
                    tunnel: [w1328] -> w1149
                    tunnel: [w1327] -> w1148
                    tunnel: [w1375] -> w1156
                    tunnel: [w1376] -> w1157
                    tunnel: w1149 -> [w1376]
                    tunnel: w1148 -> [w1375]
                    tunnel: [w1372] -> w1146
                    frame #0 {
                      w1158 = "設定5"
                      # "複製時に変更する項目\n①②③④⑤⑥⑦⑧⑨　⑪⑫\nローカル変数\n⑬⑭\nセレクション\n⑮⑯\nプロパティノードが\n対象配列になっているか確認\n⑰\n指標値\n⑱\n複製したケースのTrue定数を削除"
                      # "⑭"
                      # "⑬"
                      # "⑫"
                      # "⑪"
                      # "④"
                      # "③"
                      # "setting.iniファイルからの設定項目の読み取り"
                      n446 = local read "メイン設定No_設定 5"() -> (w1178:T5)
                      n447 = call-poly <vilib>:"Read Key.vi"("section"="No5.", "error in (no error)"=w1182, "key"="No.", "refnum"=w1181) -> ("error out"=w1175:errorcluster, "value"=w1179:i32, "refnum out"=w1173:T10)  [unwired: 4 in, 1 out]
                      n448 = Bundle By Name(cluster=w1178, "No."=w1179) -> (w1180:T5)
                      n449 = local write "メイン設定No_設定 5"(w1180) -> ()
                      n450 = for {
                        shift-right: [w1190] -> w1177
                        shift-left: w1173 -> [w1191]
                        shift-right: [w1187] -> w1176
                        shift-left: w1175 -> [w1188]
                        tunnel: string[] ["規格", "規格上限", "規格下限", "ポートNo.", "測定モード", "規格単位", "品質チェック項目", "測定周期", "実測MAX", "実測MIN", "実測(MAX)", "実測(MIN)", "測定画面表示ボタン", "ゲージポートNo."] -> [w1186] mode=indexing
                        tunnel: w1158 -> [w1183]
                        i -> [w1189]
                        # "②"
                        # "①"
                        n451 = local read "メイン設定_設定 5"() -> (w1184:T2)
                        n452 = case shown="0, デフォルト" w1189 {
                          tunnel: w1191 -> [w1200 w1209 w1218 w1227 w1236 w1245 w1254 w1263 w1272 w1281 w1290 w1299 w1308 w1317]
                          tunnel: [w1199 w1208 w1217 w1226 w1235 w1244 w1253 w1262 w1271 w1280 w1289 w1298 w1307 w1316] -> w1190
                          tunnel: w1183 -> [w1198 w1207 w1216 w1225 w1234 w1243 w1252 w1261 w1270 w1279 w1288 w1297 w1306 w1315]
                          tunnel: w1188 -> [w1197 w1206 w1215 w1224 w1233 w1242 w1251 w1260 w1269 w1278 w1287 w1296 w1305 w1314]
                          tunnel: [w1196 w1205 w1214 w1223 w1232 w1241 w1250 w1259 w1268 w1277 w1286 w1295 w1304 w1313] -> w1187
                          tunnel: w1186 -> [_ _ _ _ _ w1239 _ _ _ _ _ _ _ _]
                          tunnel: w1186 -> [_ _ _ _ _ _ w1248 _ _ _ _ w1293 _ _]
                          tunnel: w1186 -> [w1194 w1203 w1212 w1221 w1230 _ _ w1257 w1266 w1275 w1284 _ w1302 w1311]
                          tunnel: [w1193 w1202 w1211 w1220 w1229 w1237 w1246 w1255 w1265 w1274 w1283 w1292 w1301 w1310] -> w1185
                          tunnel: w1184 -> [w1192 w1201 w1210 w1219 w1228 w1238 w1247 w1256 w1264 w1273 w1282 w1291 w1300 w1309]
                          frame 0, Default {
                            n453 = call-poly <vilib>:"Read Key.vi"("section"=w1198, "error in (no error)"=w1197, "key"=w1194, "refnum"=w1200) -> ("error out"=w1196:errorcluster, "value"=w1195:string, "refnum out"=w1199:T10)  [unwired: 4 in, 1 out]
                            n454 = Bundle By Name(cluster=w1192, "規格"=w1195) -> (w1193:T2)
                          }
                          frame 1 {
                            n455 = call-poly <vilib>:"Read Key.vi"("section"=w1207, "error in (no error)"=w1206, "key"=w1203, "refnum"=w1209) -> ("error out"=w1205:errorcluster, "value"=w1204:string, "refnum out"=w1208:T10)  [unwired: 4 in, 1 out]
                            n456 = Bundle By Name(cluster=w1201, "規格上限"=w1204) -> (w1202:T2)
                          }
                          frame 2 {
                            n457 = call-poly <vilib>:"Read Key.vi"("section"=w1216, "error in (no error)"=w1215, "key"=w1212, "refnum"=w1218) -> ("error out"=w1214:errorcluster, "value"=w1213:string, "refnum out"=w1217:T10)  [unwired: 4 in, 1 out]
                            n458 = Bundle By Name(cluster=w1210, "規格下限"=w1213) -> (w1211:T2)
                          }
                          frame 3 {
                            n459 = call-poly <vilib>:"Read Key.vi"("section"=w1225, "error in (no error)"=w1224, "key"=w1221, "refnum"=w1227) -> ("error out"=w1223:errorcluster, "value"=w1222:i32, "refnum out"=w1226:T10)  [unwired: 4 in, 1 out]
                            n460 = Bundle By Name(cluster=w1219, "ポートNo."=w1222) -> (w1220:T2)
                          }
                          frame 4 {
                            n461 = call-poly <vilib>:"Read Key.vi"("section"=w1234, "error in (no error)"=w1233, "key"=w1230, "refnum"=w1236) -> ("error out"=w1232:errorcluster, "value"=w1231:i32, "refnum out"=w1235:T10)  [unwired: 4 in, 1 out]
                            n462 = Bundle By Name(cluster=w1228, "測定モード"=w1231) -> (w1229:T2)
                          }
                          frame 5 {
                            n463 = call-poly <vilib>:"Read Key.vi"("section"=w1243, "error in (no error)"=w1242, "key"=w1239, "refnum"=w1245) -> ("error out"=w1241:errorcluster, "value"=w1240:string, "refnum out"=w1244:T10)  [unwired: 4 in, 1 out]
                            n464 = Bundle By Name(cluster=w1238, "規格単位"=w1240) -> (w1237:T2)
                          }
                          frame 6 {
                            n465 = call-poly <vilib>:"Read Key.vi"("section"=w1252, "error in (no error)"=w1251, "key"=w1248, "refnum"=w1254) -> ("error out"=w1250:errorcluster, "value"=w1249:string, "refnum out"=w1253:T10)  [unwired: 4 in, 1 out]
